vi "ClusterElementNames.vi"(8 "error in":errorcluster, 11 "input cluster":variant) -> (0 "error out":errorcluster, 2 "DataTypes":T1[](array[typedef]), 3 "Elements Names":string[](array[string]), 5 "placeholder names":string[](array[string]), 7 "placeholder types":T1[](array[typedef]))   [LabVIEW 2013, in "data interface script.lvlib"]
uses:
  data interface script.lvlib
  <vilib>/NI/Tag Bus/tag/Data Type.ctl
  <vilib>/Utility/VariantDataType/Type.ctl
  <vilib>/Utility/VariantDataType/VariantType.lvlib
  <vilib>/NI/Tag Bus/tag/tag descriptor.lvclass
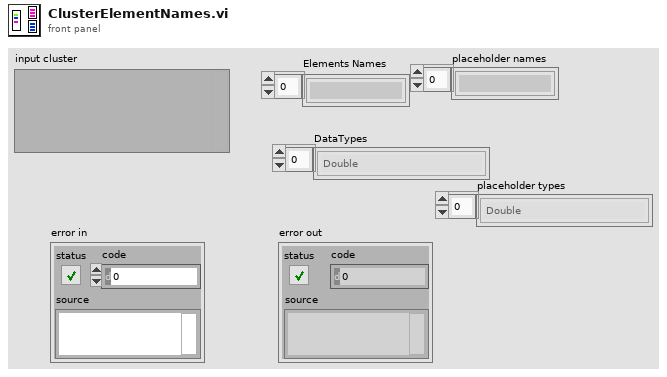
[diagram p1: front panel]
types:
  T1 = typedef "tag bus.lvlib/tag descriptor.lvclass/Data Type.ctl" = enum16{"Double", "Single", "I64", "I32", "I16", "I8", "U64", "U32", "U16", "U8", "Boolean", "String", "Array of Double", "Array of Single", "Array of I64", "Array of I32", "Array of I16", "Array of I8", "Array of U64", "Array of U32", "Array of U16", "Array of U8", "Array of Boolean", "Array of String"}
  T2 = typedef "VariantType.lvlib/Type.ctl" = enum8{"Invalid Type", "Void", "I8", "I16", "I32", "I64", "U8", "U16", "U32", "U64", "Single Float", "Double Float", "Extended Float", "Single Complex", "Double Complex", "Extended Complex", "Enum U8", "Enum U16", "Enum U32", "Enum U64", "Single Float With Unit", "Double Float With Unit", "Extended Float With Unit", "Single Complex with Unit", "Double Complex with Unit", "Extended Complex with Unit", "Boolean", "String", "Path", "Picture", "Tag", "Array", "Cluster", "Variant", "LV Variant", "Waveform", "Timestamp", "Digital Waveform", "Digital Data", "ExpressData", "Refnum", "External Data", "VI", "Poly VI", "LabVIEW Class Instance", "Fixed Point"}
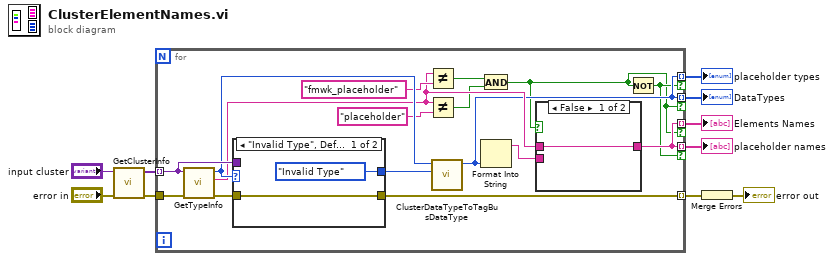
[diagram p0: block diagram]
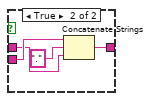
[diagram p2: hidden frame]
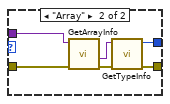
[diagram p3: hidden frame]
diagram:
  n1 = call <vilib>:"GetClusterInfo.vi"("error in (no error)"="error in", "Variant"="input cluster") -> ("error out"=w6:errorcluster, "Cluster Elements"=w9:variant[])  [unwired: 8 in]
  n2 = for {
    tunnel: w9 -> [w24] mode=indexing
    tunnel: [w13] -> w3 mode=indexing if=w11
    tunnel: [w14] -> w8 mode=indexing if=w11
    tunnel: w6 -> [w26]
    tunnel: [w20] -> w5 mode=indexing
    tunnel: [w14] -> w2 mode=indexing if=w12
    tunnel: [w13] -> w1 mode=indexing if=w12
    n3 = call <vilib>:"GetTypeInfo.vi"("error in (no error)"=w26, "Variant"=w24) -> ("error out"=w21:errorcluster, "Name"=w17:string, "Type Enum"=w22:T2)  [unwired: 5 in, 2 out]
    n4 = case shown="\"Invalid Type\", Default" w22 {
      tunnel: w24 -> [_ w39]
      tunnel: [Type."Invalid Type" ("Type Enum") w36] -> w23
      tunnel: w21 -> [w32 w35]
      tunnel: [w32 w34] -> w20
      frame "Invalid Type", Default {
      }
      frame "Array" {
        n5 = call <vilib>:"GetArrayInfo.vi"("error in (no error)"=w35, "Variant"=w39) -> ("error out"=w38:errorcluster, "ArrayElement"=w37:variant)  [unwired: 6 in, 2 out]
        n6 = call <vilib>:"GetTypeInfo.vi"("error in (no error)"=w38, "Variant"=w37) -> ("error out"=w34:errorcluster, "Type Enum"=w36:T2)  [unwired: 5 in, 3 out]
      }
    }
    n7 = Not Equal?(x=w17, y="fmwk_placeholder") -> (x != y?=w15:bool)
    n8 = Not Equal?(x=w17, y="placeholder") -> (x != y?=w16:bool)
    n9 = call "ClusterDataTypeToTagBusDataType.vi"("Array Type"=w23, "Type Enum"=w22) -> ("data type"=w13:T1)  [unwired: 9 in]
    n10 = And(x=w15, y=w16) -> (x .and. y?=w11:bool)
    n11 = Format Into String(w13) -> (resulting string=w25:string)  [unwired: 3 in, 1 out]
    n12 = case shown="False" w11 {
      tunnel: w25 -> [_ w31]
      tunnel: w17 -> [w27 w29]
      tunnel: [w27 w28] -> w14
      frame False {
      }
      frame True {
        n13 = Concatenate Strings(w31, "." ("string"), w29) -> (w28:string)
      }
    }
    n14 = Not(x=w11) -> (.not. x?=w12:bool)
  }
  "Elements Names" <- w8
  "DataTypes" <- w3
  "placeholder names" <- w2
  "placeholder types" <- w1
  n15 = Merge Errors(w5) -> (→"error out":errorcluster)
